vi "Find All Zeros of f(x).vi"   [LabVIEW 2024, in "NI_Gmath.lvlib"]
doc: "<p>Determines all zeros of a 1D function in a given interval. You must <a href=\"nihelplauncher://docs/csh?context=lvcore_lvhowto_selectingdefaultinstpolyvi\">manually select the polymorphic instance</a> to use.</p>"
uses:
  NI_Gmath.lvlib
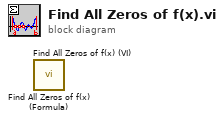
[diagram p0: block diagram]
diagram:
  n1 = call "Find All Zeros of f(x) (Formula).vi"() -> ()  [unwired: 8 in, 4 out]
  n2 = call "Find All Zeros of f(x) (VI).vi"() -> ()  [unwired: 8 in, 4 out]
